vi "Initialize.vi"(8 "error in (no error)":errorcluster, 10 "ID Query (True)":bool=TRUE, 11 "VISA resource name":refnum<visa-resource-name>) -> (0 "error out":errorcluster, 3 "VISA resource name out":refnum<visa-resource-name>)   [LabVIEW 2015, in "Siglent SPD3000 Series.lvlib"]
doc: "Establishes communication with the instrument and optionally performs an instrument identification query and/or an instrument reset. It also places the instrument in a default state needed for other instrument driver operations. Therefore, call this VI before calling other instrument driver VIs for this instrument. Generally, you need to call the Initialize VI only once at the beginning of an application."
uses:
  <instrlib>/Siglent SPD3000 Series/Siglent SPD3000 Series.lvlib
panel:
  # "(c) 2016 SIGLENT TECHNOLOGIES CO., LTD.   ALL RIGHTS RESERVED."
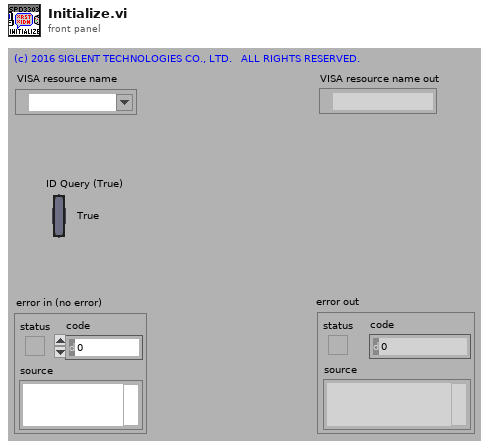
[diagram p1: front panel]
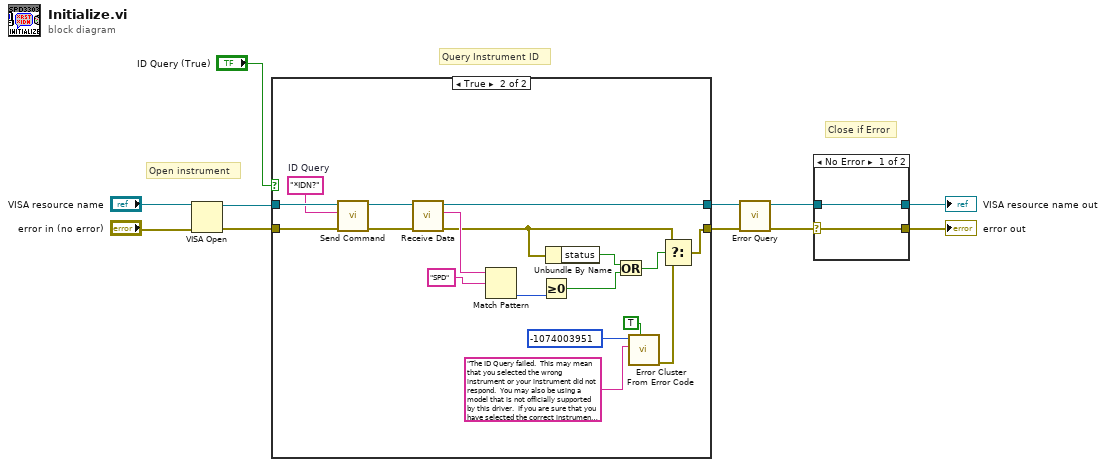
[diagram p0: block diagram]
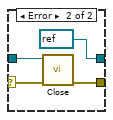
[diagram p2: hidden frame]
diagram:
  # "Close if Error"
  # "Query Instrument ID"
  # "Open instrument"
  n1 = VISA Open(error in (no error)="error in (no error)", VISA resource name="VISA resource name") -> (VISA resource name=w3:refnum<visa-resource-name>, error out=w2:errorcluster)  [unwired: 3 in]
  n2 = case shown="True" "ID Query (True)" {
    tunnel: [w12 w31] -> w8
    tunnel: [w13 w28] -> w7
    tunnel: w3 -> [w13 w29]
    tunnel: w2 -> [w12 w30]
    frame False {
    }
    frame True {
      w25 = "*IDN?"  # ID Query
      n3 = call <instrlib>:"Send Command.vi"("error in (no error)"=w30, "Write Buffer (\"\")"=w25, "VISA resource name"=w29) -> ("error out"=w14:errorcluster, "VISA resource name out"=w15:refnum<visa-resource-name>)  [unwired: 7 in]
      n4 = call <instrlib>:"Receive Data.vi"("error in (no error)"=w14, "VISA resource name"=w15) -> ("error out"=w19:errorcluster, "Read Buffer"=w27:string, "VISA resource name out"=w28:refnum<visa-resource-name>)  [unwired: 6 in, 1 out]
      n5 = Match Pattern(string=w27, regular expression="SPD") -> (offset past match=w20:i32)  [unwired: 1 in, 3 out]
      n6 = Greater Or Equal To 0?(x=w20) -> (x >= 0?=w17:bool)
      n7 = Unbundle By Name(w19) -> ("status"=w18:bool)
      n8 = Or(x=w18, y=w17) -> (x .or. y?=w16:bool)
      n9 = call <vilib>:"Error Cluster From Error Code.vi"("show call chain? (False)"=TRUE, "error message (\"\")"="The ID Query failed.  This may mean that you selected the wrong instrument or your instrument did not respond.  You may also be using a model that is not officially supported by this driver.  If you are sure that you have selected the correct instrument and it is responding, try disabling the ID Query." ("Source (VI Name)"), "error code (0)"=-1074003951 ("Code")) -> ("error out"=w24:errorcluster)  [unwired: 6 in]
      n10 = Select(t=w19, s=w16, f=w24) -> (s? t:f=w31:errorcluster)
    }
  }
  n11 = call <instrlib>:"Error Query.vi"("error in (no error)"=w8, "VISA resource name"=w7) -> ("error out"=w5:errorcluster, "VISA resource name out"=w6:refnum<visa-resource-name>)  [unwired: 6 in, 2 out]
  n12 = case shown="No Error" w5 {
    selector: w5 -> [w32 w35]
    tunnel: w6 -> [w33 w36]
    tunnel: [w33 refnum<visa-resource-name> refnum ("VISA resource name out")] -> w10
    tunnel: [w32 w37] -> w9
    frame No Error {
    }
    frame Error {
      n13 = call <instrlib>:"Close.vi"("error in (no error)"=w35, "VISA resource name"=w36) -> ("error out"=w37:errorcluster)  [unwired: 9 in]
    }
  }
  "VISA resource name out" <- w10
  "error out" <- w9
